vi "AbortAndRunVI.vi"(8 "error out":errorcluster, 11 "appended path":path) -> (0 "error out 4":errorcluster, 3 "vi reference 4":refnum<vi>)   [LabVIEW 2015]
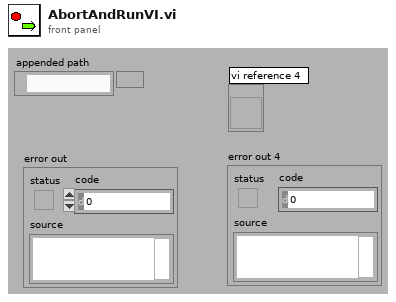
[diagram p1: front panel]
types:
  T1 = enum32{"Invalid", "Standard", "Closed", "Hidden", "Minimized", "Maximized"}
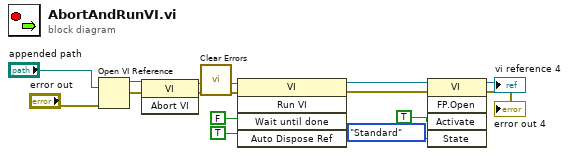
[diagram p0: block diagram]
diagram:
  n1 = Open VI Reference(vi path="appended path", error in (no error)="error out") -> (vi reference=w5:refnum<vi>, error out=w4:errorcluster)  [unwired: 4 out]
  n2 = invoke class="VI" method="Abort VI"(reference=w5, error in=w4) -> (reference out=w9:refnum<vi>, error out=w8:errorcluster)  [unwired: 1 in, 1 out]
  n3 = call <vilib>:"Clear Errors.vi"("error in (no error)"=w8) -> ("error out"=w1:errorcluster)  [unwired: 1 in, 5 out]
  n4 = invoke class="VI" method="Run VI"(reference=w9, error in=w1, "Wait until done"=FALSE ("Wait Until Done"), "Auto Dispose Ref"=TRUE ("Auto Dispose Reference")) -> (reference out=w7:refnum<vi>, error out=w6:errorcluster)  [unwired: 1 in, 3 out]
  n5 = invoke class="VI" method="FP.Open"(reference=w7, error in=w6, "Activate"=TRUE ("Activate?"), "State"=T1."Standard") -> (reference out=→"vi reference 4":refnum<vi>, error out=→"error out 4":errorcluster)  [unwired: 1 in, 3 out]
